vi "Periodic Tasks.vi"(8 "error in":errorcluster) -> ()   [LabVIEW 2023]
doc: "This VI runs in parallel to other tasks. It can contain as many user-defined periodic loops as you need. These can carry out PID or other sorts of timed response."
uses:
  <vilib>/Rock Robotics/WPI/Utilities/WPI_GetSetVariantRefNum.vi
  Robot Global Data.vi
panel:
  out "Numeric 6":dbl
  out "Numeric 5":dbl
  out "Numeric 4":dbl
  out "Numeric 3":dbl
  out "Numeric 2":dbl
  out "Numeric":dbl
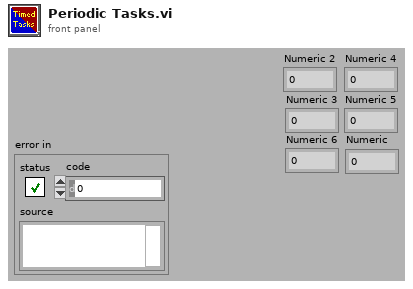
[diagram p1: front panel]
types:
  T1 = typedef "WPI_JoystickDevRef.ctl" = cluster{"Device":T2}
  T2 = typedef "WPI_JoystickDeviceEnum.ctl" = enum16{"USB 0", "USB 1", "USB 2", "USB 3", "USB 4", "USB 5"}
  T3 = typedef "WPI_RobotDriveDevRef.ctl" = cluster{"DevStatus":errorcluster, "Motors[]":T4[], "Square Inputs":bool, "Max Output":dbl}
  T4 = typedef "WPI_MotorControlDeviceRef.ctl" = cluster{"DeviceStatus":errorcluster, "Type":T5, "PWM":cluster{"PWM Channel":T6, "DeadBand":T7}, "CAN":cluster{"Device Number":u8, "SetOutput VI Ref":variant, "GetOutput VI Ref":variant, "Enable VI Ref":variant, "Disable VI Ref":variant, "Data":variant}, "Invert":bool, "DIO PWM":cluster{"PWM \"Enable\" Channel":T6, "DIOChannel":T8, "PWM Rate":dbl}}
  T5 = typedef "WPI_MotorControlType.ctl" = enum16{"PWM", "CAN", "DIO PWM"}
  T6 = typedef "FPGA_DIOPWMChannel.ctl" = enum8{"PWM 0", "PWM 1", "PWM 2", "PWM 3", "PWM 4", "PWM 5", "PWM 6", "PWM 7", "PWM 8", "PWM 9", "PWM MXP 0", "PWM MXP 1", "PWM MXP 2", "PWM MXP 3", "PWM MXP 4", "PWM MXP 5", "PWM MXP 6", "PWM MXP 7", "PWM MXP 8", "PWM MXP 9", "Invalid"}
  T7 = typedef "WPI_PWMDeadband.ctl" = cluster{"Name":string, "maxPositivePwm":i32, "minPositivePwm":i32, "centerPwm":i32, "maxNegativePwm":i32, "minNegativePwm":i32, "angularRange":u16}
  T8 = typedef "FPGA_DIOChannel.ctl" = enum8{"DIO 0", "DIO 1", "DIO 2", "DIO 3", "DIO 4", "DIO 5", "DIO 6", "DIO 7", "DIO 8", "DIO 9", "DIO MXP 0", "DIO MXP 1", "DIO MXP 2", "DIO MXP 3", "DIO MXP 4", "DIO MXP 5", "DIO MXP 6", "DIO MXP 7", "DIO MXP 8", "DIO MXP 9", "DIO MXP 10", "DIO MXP 11", "DIO MXP 12", "DIO MXP 13", "DIO MXP 14", "DIO MXP 15", "SPI Port CS1", "SPI Port CS2", "SPI Port CS3", "SPI Port MISO", "SPI Port MOSI", "Invalid"}
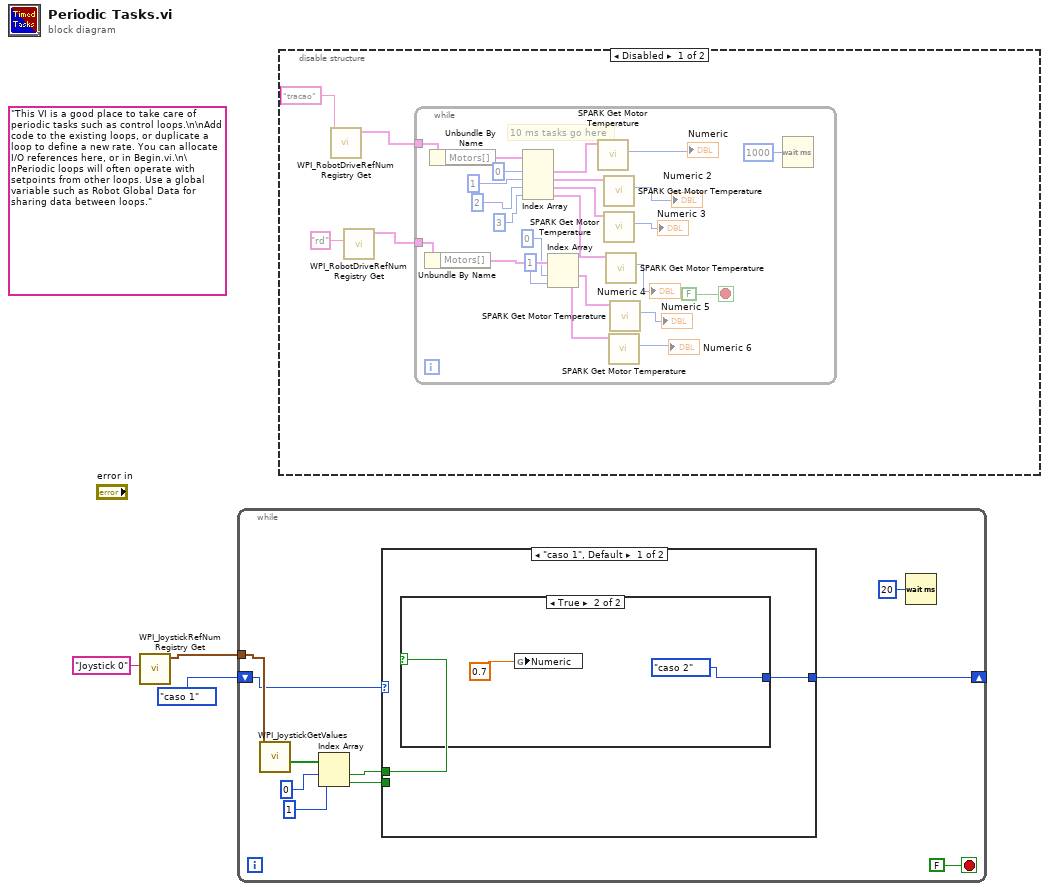
[diagram p0: block diagram]
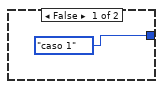
[diagram p2: hidden frame]
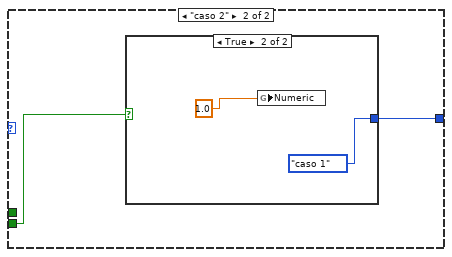
[diagram p3: hidden frame]
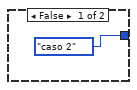
[diagram p4: hidden frame]
diagram:
  (unwired) "This VI is a good place to take care of periodic tasks such as control loops.\n\nAdd code to the existing loops, or duplicate a loop to define a new rate. You can allocate I/O references here, or in Begin.vi.\n\nPeriodic loops will often operate with setpoints from other loops. Use a global variable such as Robot Global Data for sharing data between loops."
  n1 = call <vilib>:"WPI_JoystickRefNum Registry Get.vi"("refnum name"="Joystick 0") -> ("JoystickDevRef"=w2:T1)  [unwired: 9 in, 1 out]
  n2 = while {
    tunnel: w2 -> [w12]
    shift-right: [w5] -> _
    shift-left: enum16{"caso 1", "caso 2"}."caso 1" -> [w8]
    stop <- FALSE stop-if-true
    n3 = call <vilib>:"WPI_JoystickGetValues.vi"("JoystickDevRef"=w12) -> ("Buttons"=w11:bool[])  [unwired: 6 in, 4 out]
    n4 = Index Array(array=w11, index #1=0 ("index"), index #2=1 ("index")) -> (element #1=w7:bool, element #2=w6:bool)
    n5 = case shown="\"caso 1\", Default" w8 {
      tunnel: w7 -> [w15 _]
      tunnel: w6 -> [_ w20]
      tunnel: [w14 w19] -> w5
      frame "caso 1", Default {
        n6 = case shown="True" w15 {
          tunnel: [enum16{"caso 1", "caso 2"}."caso 1" enum16{"caso 1", "caso 2"}."caso 2"] -> w14
          frame False {
          }
          frame True {
            n7 = global write "Robot Global Data.vi" "Numeric"(0.7) -> ()
          }
        }
      }
      frame "caso 2" {
        n8 = case shown="True" w20 {
          tunnel: [enum16{"caso 1", "caso 2"}."caso 2" enum16{"caso 1", "caso 2"}."caso 1"] -> w19
          frame False {
          }
          frame True {
            n9 = global write "Robot Global Data.vi" "Numeric"(1.0) -> ()
          }
        }
      }
    }
    n10 = Wait (ms)(milliseconds to wait=u32 20) -> ()  [unwired: 1 out]
  }
  n11 = disable-structure shown="Disabled" {
    frame Disabled {
      n12 = call <vilib>:"WPI_RobotDriveRefNum Registry Get.vi"("refnum name"="tracao") -> ("RobotDriveDevRef"=w26:T3)  [unwired: 9 in, 1 out]
      n13 = call <vilib>:"WPI_RobotDriveRefNum Registry Get.vi"("refnum name"="rd") -> ("RobotDriveDevRef"=w24:T3)  [unwired: 9 in, 1 out]
      n14 = while {
        tunnel: w26 -> [w49]
        tunnel: w24 -> [w47]
        stop <- FALSE stop-if-true
        # "10 ms tasks go here"
        n15 = Unbundle By Name(w47) -> ("Motors[]"=w46:T4[])
        n16 = Unbundle By Name(w49) -> ("Motors[]"=w48:T4[])
        n17 = Index Array(array=w48, index #1=0 ("index"), index #2=1 ("index"), index #3=2 ("index"), index #4=3 ("index")) -> (element #1=w39:T4, element #2=w38:T4, element #3=w37:T4, element #4=w36:T4)
        n18 = Index Array(array=w46, index #1=0 ("index"), index #2=1 ("index")) -> (element #1=w31:T4, element #2=w30:T4)
        n19 = call <vilib>:"SPARK Get Motor Temperature.vi"("MotorControlDevRef in"=w39) -> ("Motor Temperature"=→"Numeric":u8)  [unwired: 7 in, 3 out]
        n20 = call <vilib>:"SPARK Get Motor Temperature.vi"("MotorControlDevRef in"=w38) -> ("Motor Temperature"=→"Numeric 2":u8)  [unwired: 7 in, 3 out]
        n21 = call <vilib>:"SPARK Get Motor Temperature.vi"("MotorControlDevRef in"=w37) -> ("Motor Temperature"=→"Numeric 3":u8)  [unwired: 7 in, 3 out]
        n22 = call <vilib>:"SPARK Get Motor Temperature.vi"("MotorControlDevRef in"=w36) -> ("Motor Temperature"=→"Numeric 4":u8)  [unwired: 7 in, 3 out]
        n23 = call <vilib>:"SPARK Get Motor Temperature.vi"("MotorControlDevRef in"=w30) -> ("Motor Temperature"=→"Numeric 6":u8)  [unwired: 7 in, 3 out]
        n24 = call <vilib>:"SPARK Get Motor Temperature.vi"("MotorControlDevRef in"=w31) -> ("Motor Temperature"=→"Numeric 5":u8)  [unwired: 7 in, 3 out]
        n25 = Wait (ms)(milliseconds to wait=u32 1000) -> ()  [unwired: 1 out]
      }
    }
    frame Enabled {
    }
  }
